vi "Append Text To Document Word.vi"() -> ()   [LabVIEW 2017]
doc: "Demonstrates how to add formatted texts to an MS Word document."
uses:
  LabVIEW NPOI/Document/Document.lvclass/Document.ctl
  LabVIEW NPOI/Document/Get FilePath.vi
  LabVIEW NPOI/Document/Document.lvclass
panel:
  in  "Paragraph":string="Lorem ipsum dolor sit amet, consectetur adipiscing elit, sed do eiusmod tempor incididunt ut labore et dolore magna aliqua. Adipiscing bibendum est ultricies integer quis auctor elit sed vulputate. Volutpat consequat mauris nunc congue nisi vitae suscipit tellus. Eget arcu dictum varius duis at consectetur lorem donec massa. Morbi enim nunc faucibus a pellentesque sit. Risus ultricies tristique nulla aliquet enim tortor at. Sit amet consectetur adipiscing elit ut aliquam purus sit. Porta lorem mollis aliquam ut porttitor leo a diam. Odio aenean sed adipiscing diam donec adipiscing tristique risus. Nunc eget lorem dolor sed viverra ipsum nunc aliquet. Ultrices gravida dictum fusce ut. Mi eget mauris pharetra et ultrices. Ultrices dui sapien eget mi proin. Duis ut diam quam nulla porttitor massa id neque. Eu lobortis elementum nibh tellus molestie nunc non. Iaculis nunc sed augue lacus viverra. Enim sed faucibus turpis in eu. Quis viverra nibh cras pulvinar mattis. Auctor augue mauris augue neque gravida. Enim ut tellus elementum sagittis vitae."
  in  "Sub-Title":string="Lorem ipsum sub-title"
  out "File Path":path
  in  "Document Format":enum16{"xlsx", "xls", "docx", "doc"}(ring)=enum."docx"
  in  "Title":string="Lorem Ipsum Document"
  # "Overview: Demonstrates how to add formatted texts to an MS Word document.\nInstructions:\n1. Select the Document Format you want to create.\n        Optionally: You can change the Title, the Sub-Title and the Paragraph.\n2. Run the VI.\n3. The generated document will be located at the path indicated by File Path.\n4. Delete the temporary Document file when you are done."
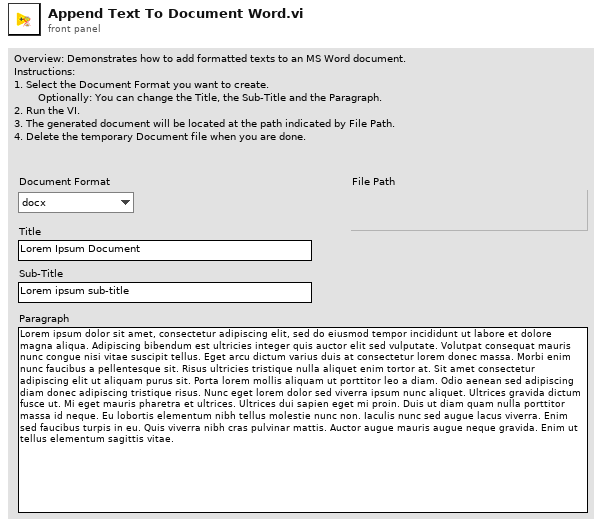
[diagram p1: front panel]
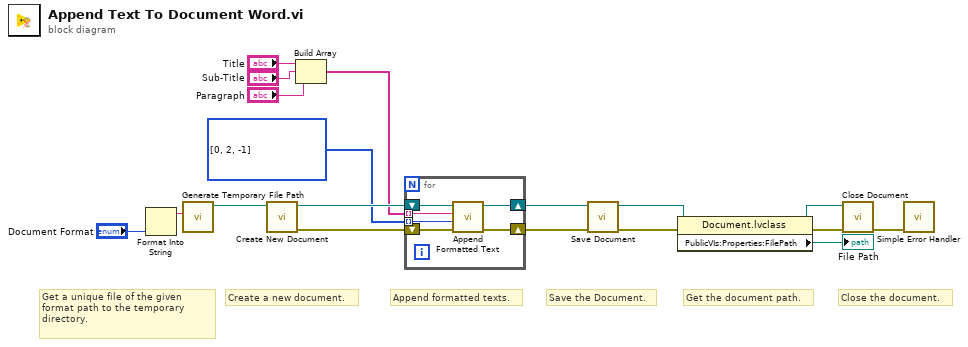
[diagram p0: block diagram]
diagram:
  w1 = i32[] [0, 2, -1] items=["Title"=0, "H1"=1, "H2"=2, "H3"=3, "H4"=4, "Paragraph"=-1] ("Heading Level (-1)")
  # "Close the document."
  # "Get the document path."
  # "Save the Document."
  # "Append formatted texts."
  # "Create a new document."
  # "Get a unique file of the given format path to the temporary directory."
  n1 = Format Into String("Document Format") -> (resulting string=w10:string)  [unwired: 3 in, 1 out]
  n2 = call <vilib>:"Generate Temporary File Path.vi"("Temporary File Extension (tmp)"=w10) -> ("Unique Temporary File Path"=w9:path)  [unwired: 9 in, 1 out]
  n3 = call "Create New Document.vi"("File Path"=w9) -> ("error out"=w18:errorcluster, "Document out"=w8:refnum<class "Document.lvclass">)  [unwired: 9 in]
  n4 = Build Array("Title", "Sub-Title", "Paragraph") -> (w2:string[])
  n5 = for {
    shift-right: [w21] -> w6
    shift-left: w18 -> [w24]
    shift-right: [w22] -> w7
    shift-left: w8 -> [w23]
    tunnel: w2 -> [w20] mode=indexing
    tunnel: w1 -> [w19] mode=indexing
    n6 = call "Append Formatted Text.vi"("error in (no error)"=w24, "Heading Level (-1)"=w19, "Heading Text"=w20, "Document in"=w23) -> ("error out"=w21:errorcluster, "Document out"=w22:refnum<class "Document.lvclass">)  [unwired: 6 in]
  }
  n7 = call "Save Document.vi"("error in (no error)"=w6, "Document in"=w7) -> ("error out"=w14:errorcluster, "Document out"=w17:refnum<class "Document.lvclass">)  [unwired: 8 in]
  n8 = property class="Document.lvclass"(reference=w17, error in=w14) -> (reference out=w15:refnum<class "Document.lvclass">, error out=w13:errorcluster, "PublicVIs:Properties:FilePath"=→"File Path":path)
  n9 = call "Close Document.vi"("error in (no error)"=w13, "Document in"=w15) -> ("error out"=w16:errorcluster)  [unwired: 9 in]
  n10 = call <vilib>:"Simple Error Handler.vi"("error in (no error)"=w16) -> ()  [unwired: 4 in, 5 out]
